vi "BRig_RT_panel_Laser1_DAB_v1,10.vi"(7 "input_setValues":bool, 9 "input_dataExp":u16[](array[numeric]), 11 "input_dataLC":u16[](array[numeric])) -> (1 "output_dataExp":u16[](array[numeric]), 3 "output_dataLC":u16[](array[numeric]))   [LabVIEW 2014]
panel:
  out "LaserPulseTrain":cluster{u16[], u16[]}(graph)
  in  "LED_baseline":bool
  in  "Laser_power_step":dbl
  in  "Laser_power_max":dbl
  in  "Laser_power_min":dbl
  in  "Laser_Tshutter":u16=2
  in  "Laser_Freq":u16=10
  in  "Laser_Tpeak":u16=2
  in  "Laser_T":u16
  in  "LC_Sel_First_Count":u16
  in  "LC_Sel_First_Probability":u16
  in  "LC_Sel_First_Block":u16(slide) max=2 step=1 scale=0.0..2.0
  in  "LC_Sel_First_OnOff":bool
  in  "LC_Sel_First_Tdelay":u16
  in  "LC_Cue_First_Count":u16
  in  "LC_ENL_First_Count":u16
  in  "LC_Cue_First_delayOpt":bool
  in  "LC_ENL_First_delayOpt":bool
  in  "LC_Reward_Probability":u16
  in  "LC_Reward_Block":u16(slide) max=2 step=1 scale=0.0..2.0
  in  "LC_Reward_OnOff":bool
  in  "LC_Cue_First_Probability":u16
  in  "LC_Cue_First_Block":u16(slide) max=2 step=1 scale=0.0..2.0
  in  "LC_Cue_First_OnOff":bool
  in  "LC_ENL_First_Probability":u16 max=100 step=1
  in  "LC_ENL_First_Block":u16(slide) max=2 step=1 scale=0.0..2.0
  in  "LC_Reward_Tdelay":u16
  in  "LC_Cue_First_Tdelay":u16
  in  "LC_ENL_First_Tdelay":u16
  in  "LC_ENL_First_OnOff":bool
  # "Laser1 Control\n                               On/Off      Block        Probability [%]   Delay [ms]                              Count"
  # "Enforced\nNonLick"
  # "from end"
  # "from start"
  # "Cue"
  # "from end"
  # "from start"
  # "Selection"
  # "from start"
  # "Laser1 Parameters"
  # "Laser1 Response\n           On/Off      Response                 Probability %  Delay [ms]"
  # "Frequency\n[Hz]"
  # "Selection\nReward"
  # "Timing [ms]\n Duration     Peak Width   Shutter"
  # "If flip event (reward amount and probability get flipped)\nthen adjust the response setting as well (e.g. Left->Right)"
  # "Laser Power [V]\nMin          Max              Step"
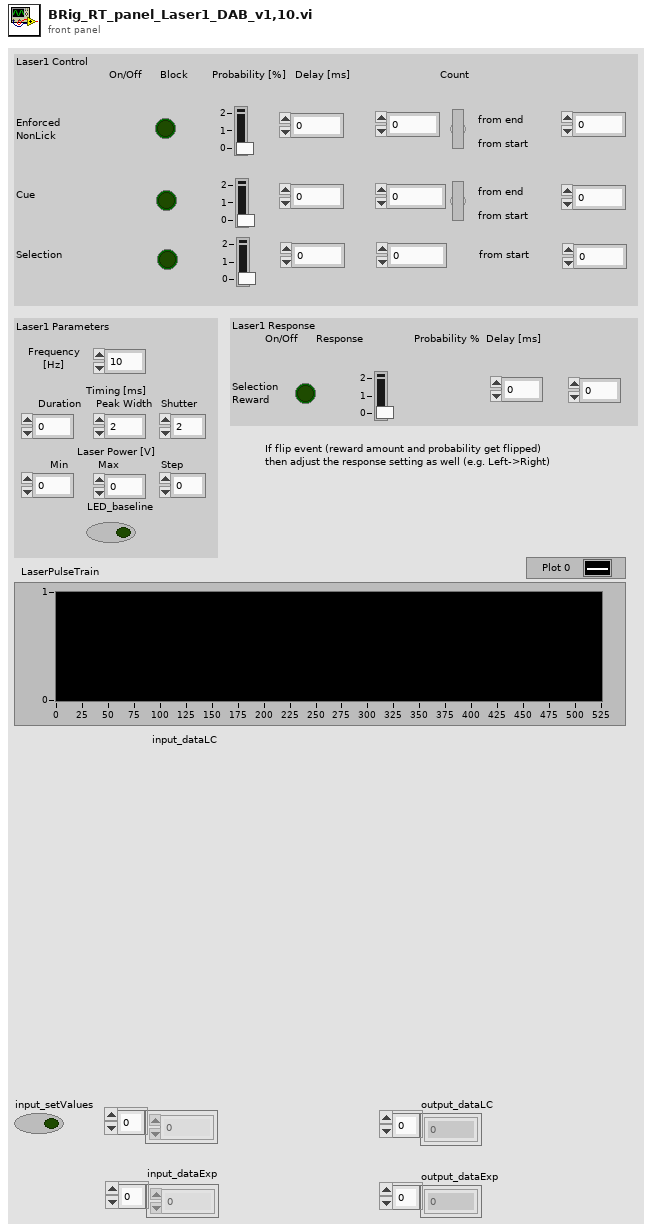
[diagram p1: front panel]
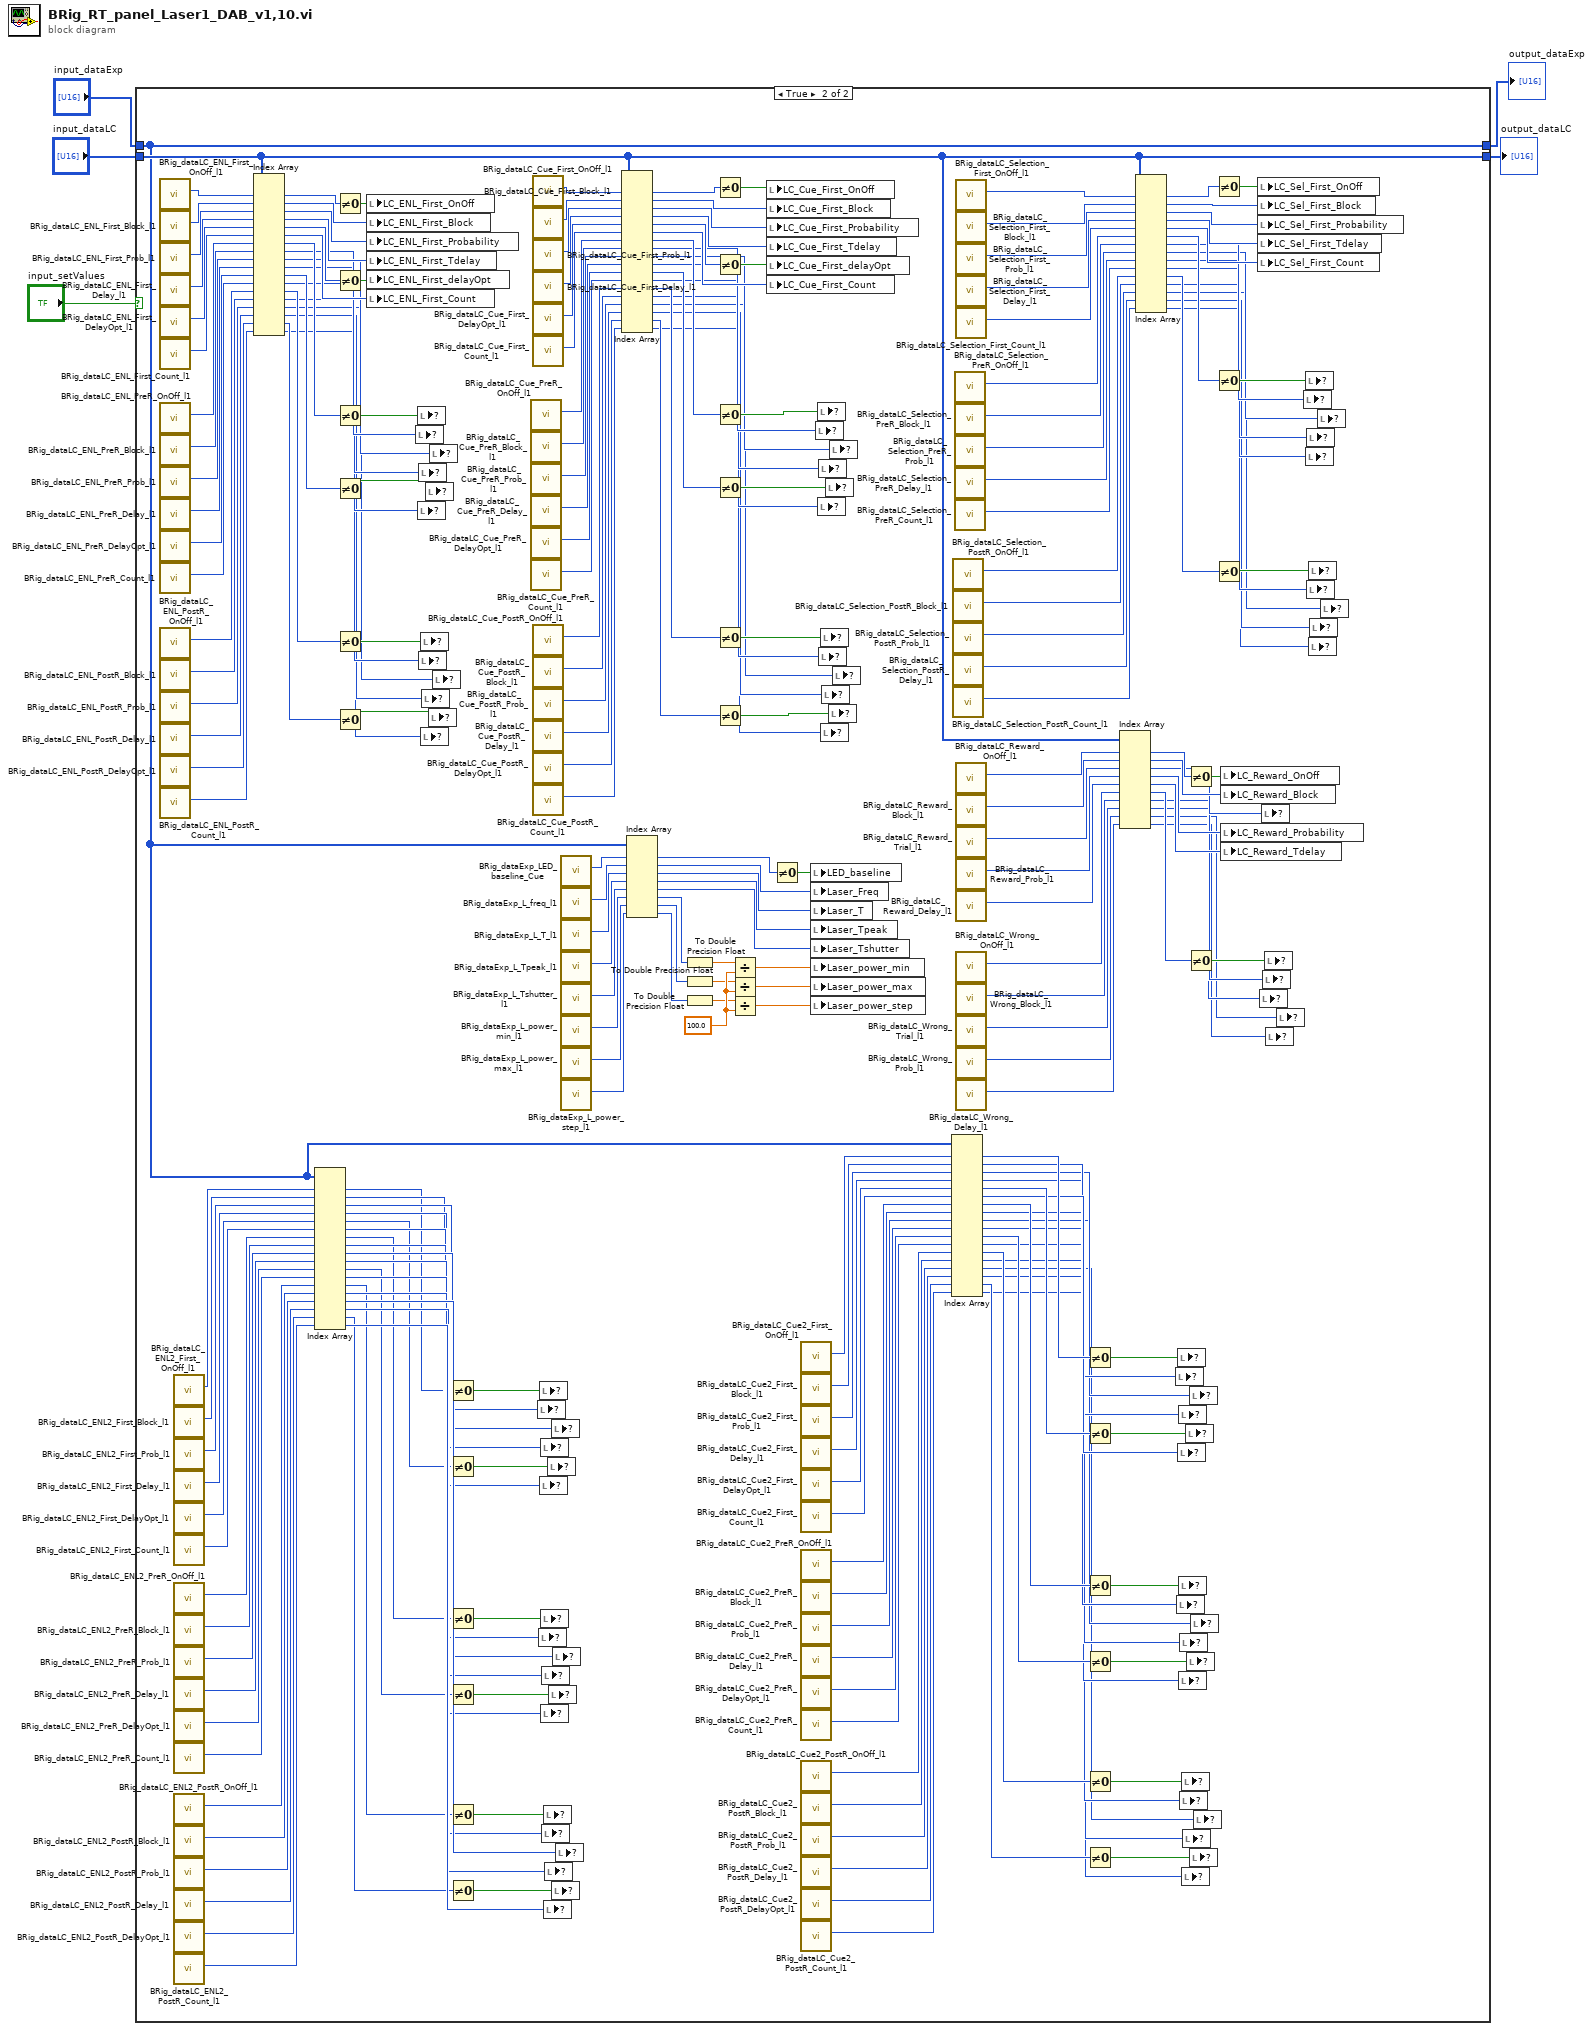
[diagram p0: block diagram]
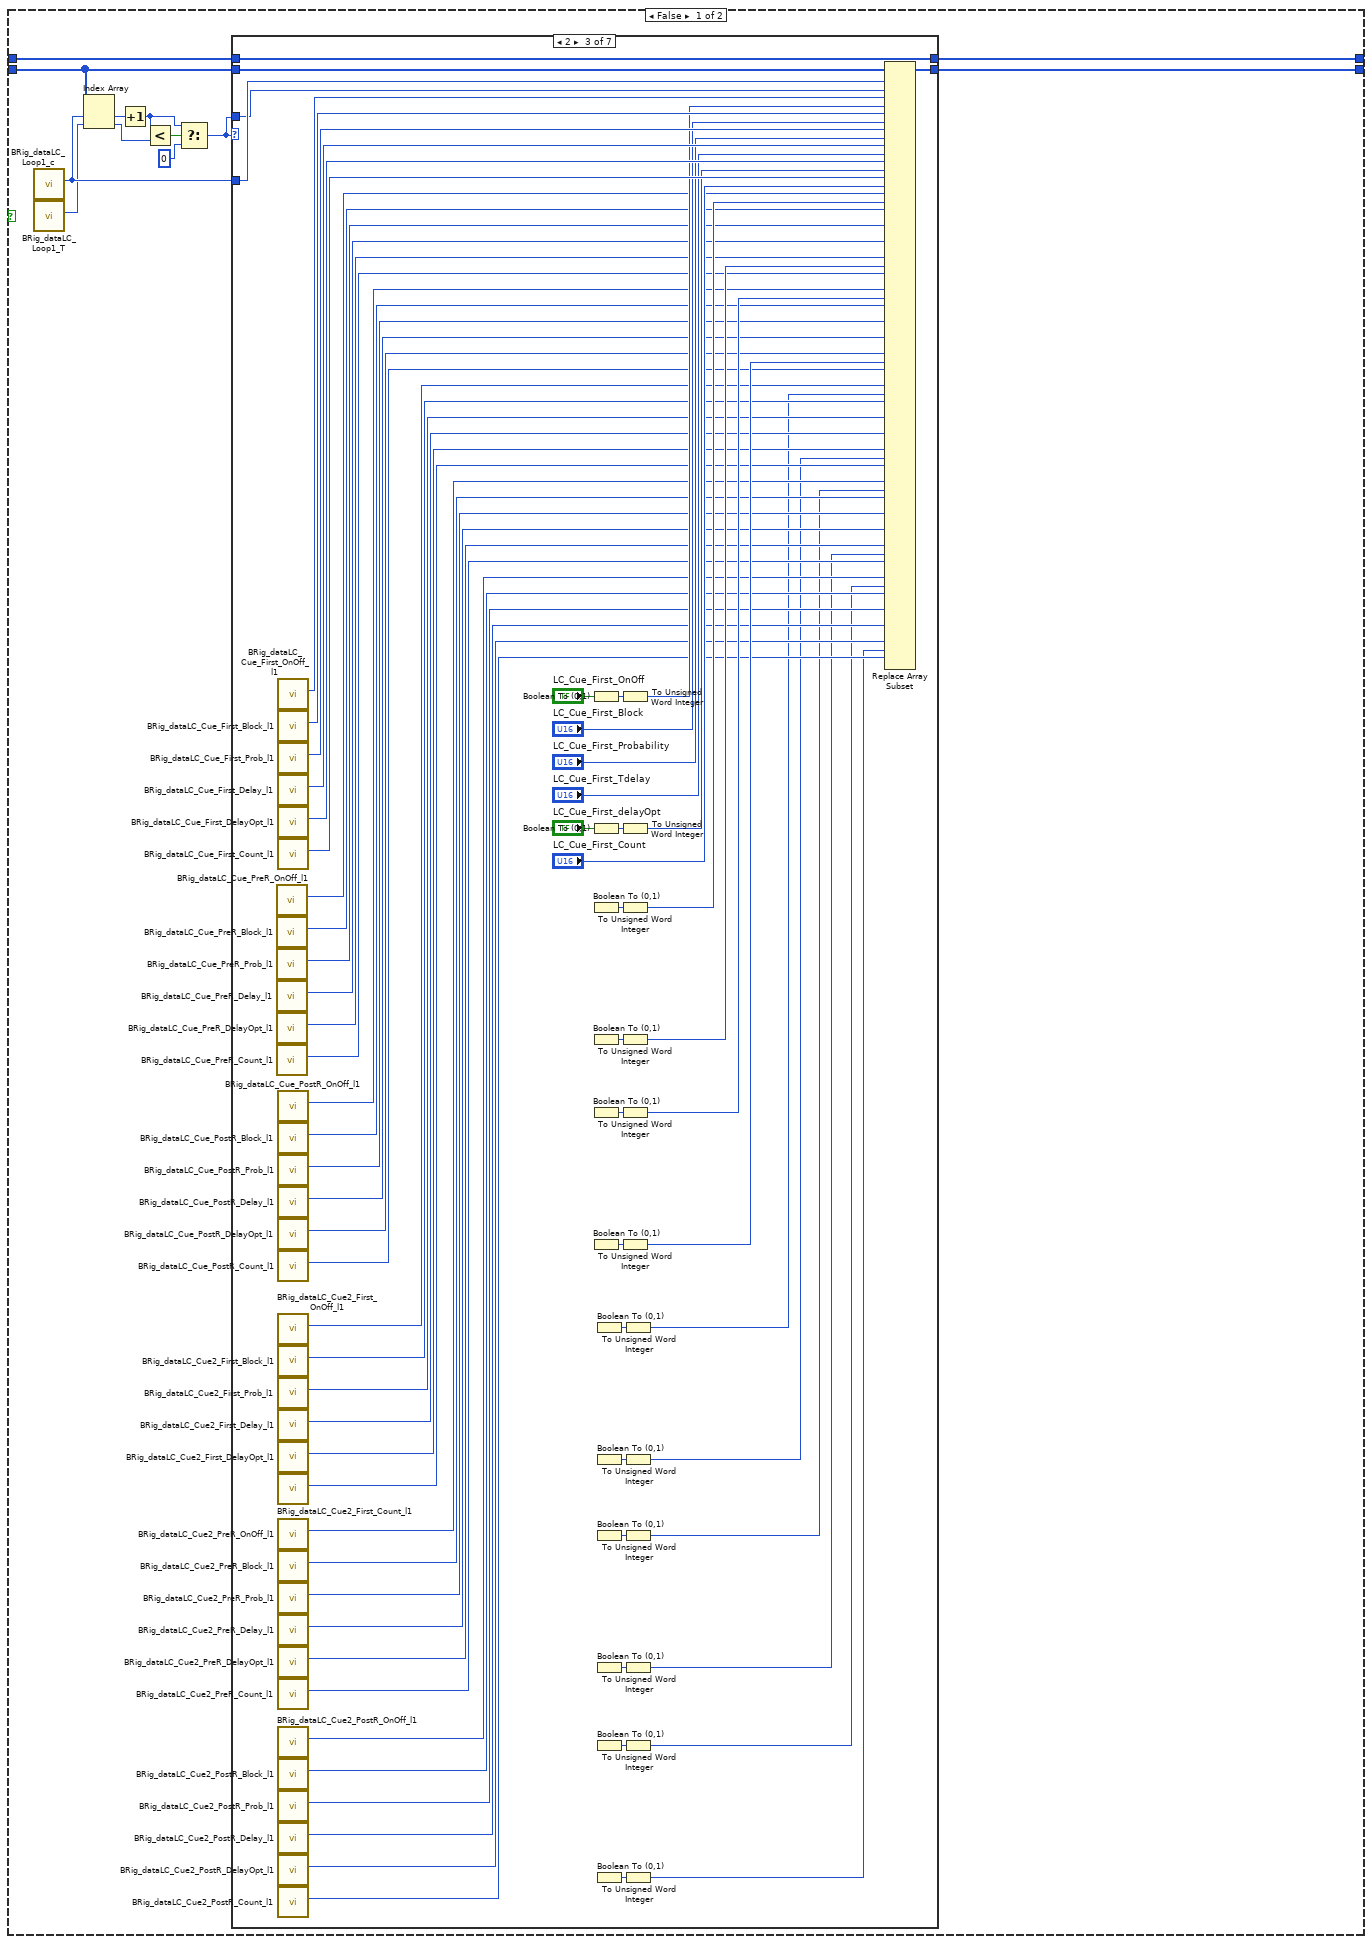
[diagram p2: hidden frame]
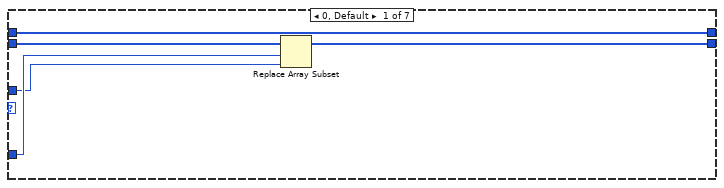
[diagram p3: hidden frame]
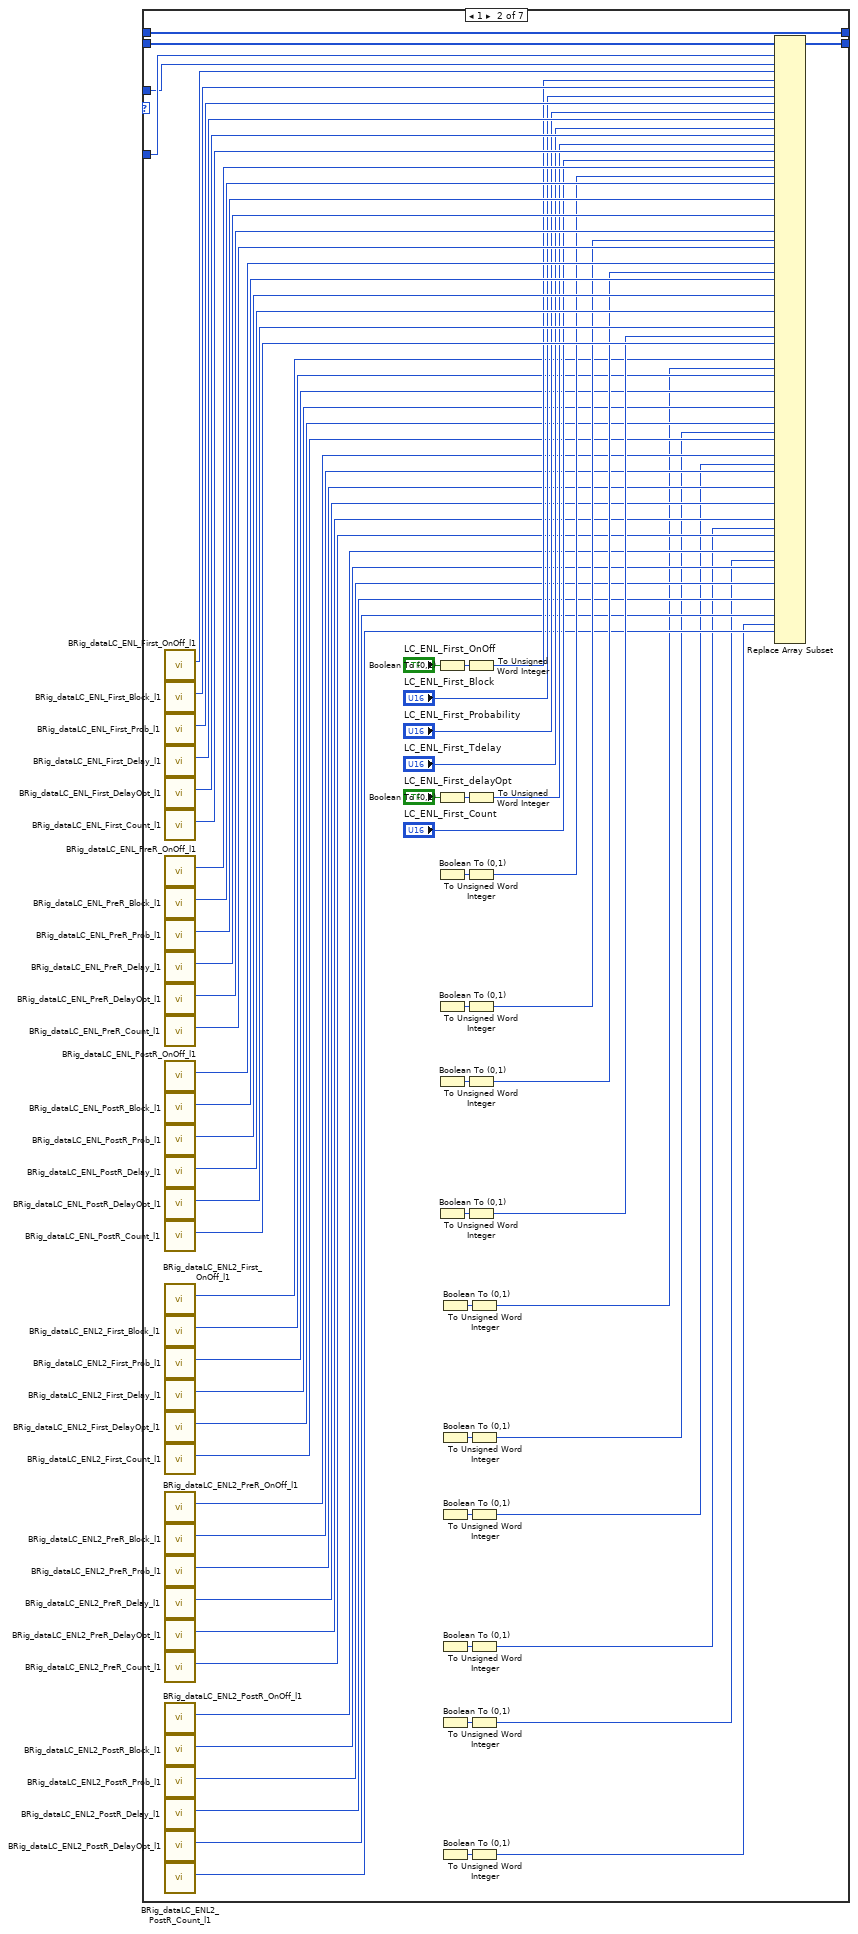
[diagram p4: hidden frame]
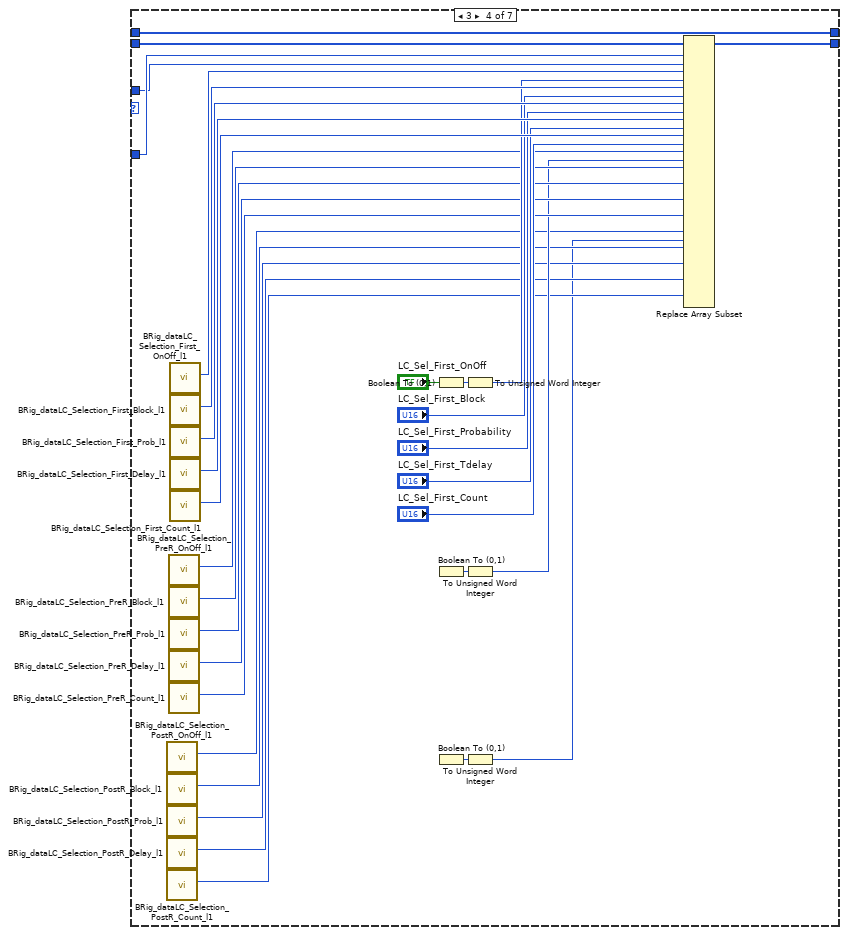
[diagram p5: hidden frame]
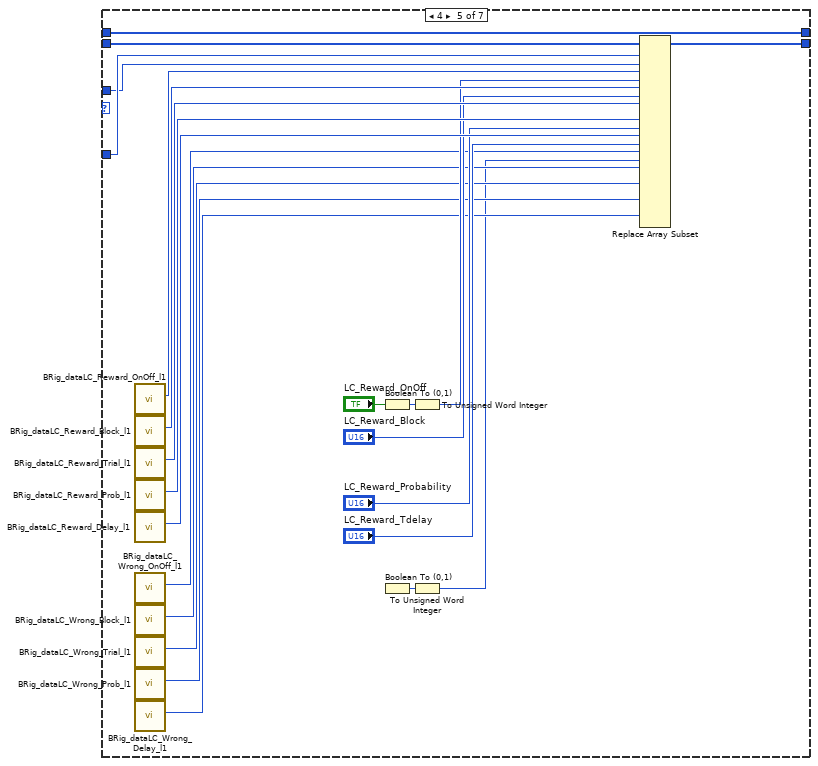
[diagram p6: hidden frame]
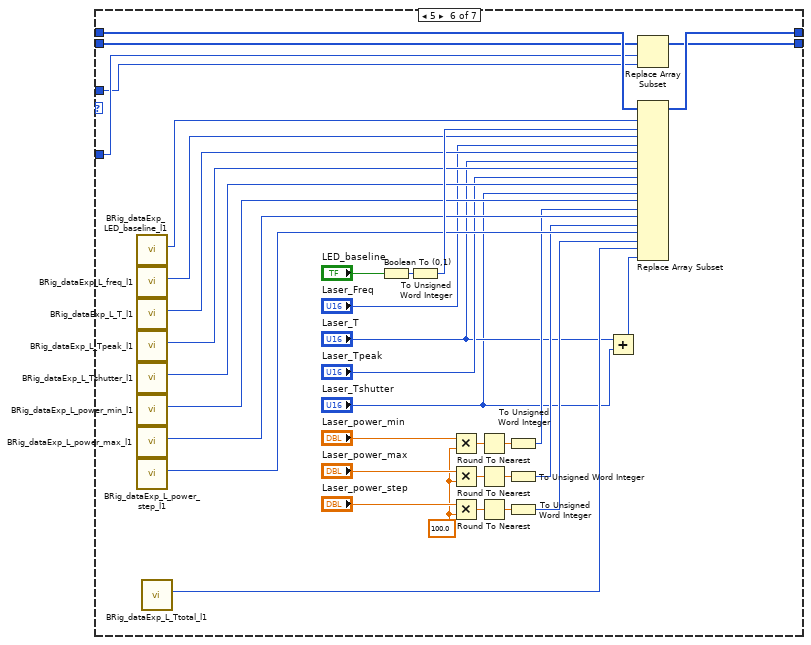
[diagram p7: hidden frame]
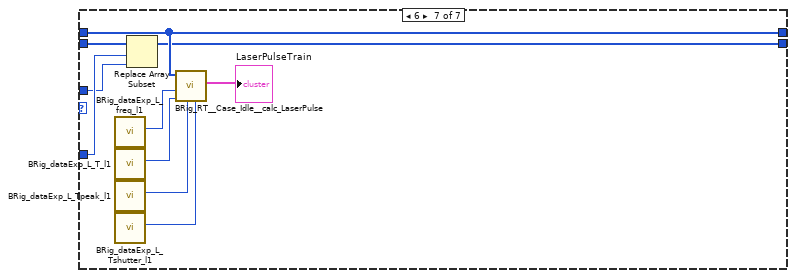
[diagram p8: hidden frame]
diagram:
  n1 = case shown="True" "input_setValues" {
    tunnel: "input_dataLC" -> [w17 w445]
    tunnel: [w11 w445] -> w4
    tunnel: "input_dataExp" -> [w7 w360]
    tunnel: [w6 w360] -> w1
    frame False {
      n2 = call "BRig_dataLC_Loop1_c.vi"() -> ("output_Loop1_c"=w10:i32)  [unwired: 11 in]
      n3 = call "BRig_dataLC_Loop1_T.vi"() -> ("output_Loop1_T"=w9:i32)  [unwired: 11 in]
      n4 = Index Array(array=w17, index #1=w10, index #2=w9) -> (element #1=w16:u16, element #2=w15:u16)
      n5 = Increment(x=w16) -> (x+1=w12:u16)
      n6 = Less?(x=w12, y=w15) -> (x < y?=w14:bool)
      n7 = Select(t=w12, s=w14, f=u16 0) -> (s? t:f=w8:u16)
      n8 = case shown="2" w8 {
        tunnel: w17 -> [w22 w113 w210 w249 w277 w282 w321]
        tunnel: w10 -> [w20 w67 w176 w213 w252 w280 w319]
        tunnel: w8 -> [w19 w66 w175 w212 w251 w279 w318]
        tunnel: [w21 w106 w209 w248 w276 w281 w320] -> w11
        tunnel: w7 -> [w18 w65 w162 w211 w250 w284 w323]
        tunnel: [w18 w65 w162 w211 w250 w283 w323] -> w6
        frame 0, Default {
          n9 = Replace Array Subset(array=w22, new element=w19, index=w20) -> (w21:u16[])
        }
        frame 1 {
          n10 = call "BRig_dataLC_ENL_First_OnOff_l1.vi"() -> ("output_ENL_First_OnOff"=w112:i32)  [unwired: 11 in]
          n11 = call "BRig_dataLC_ENL_First_Block_l1.vi"() -> ("output_ENL_First_Block"=w111:i32)  [unwired: 11 in]
          n12 = call "BRig_dataLC_ENL_First_Prob_l1.vi"() -> ("output_ENL_First_Prob"=w110:i32)  [unwired: 11 in]
          n13 = call "BRig_dataLC_ENL_First_Delay_l1.vi"() -> ("output_ENL_First_Delay"=w109:i32)  [unwired: 11 in]
          n14 = call "BRig_dataLC_ENL_First_DelayOpt_l1.vi"() -> ("output_ENL_First_DelayOpt"=w108:i32)  [unwired: 11 in]
          n15 = call "BRig_dataLC_ENL_First_Count_l1.vi"() -> ("output_ENL_First_Count"=w107:i32)  [unwired: 11 in]
          n16 = call "BRig_dataLC_ENL_PreR_OnOff_l1.vi"() -> ("output_ENL_PreR_OnOff"=w105:i32)  [unwired: 11 in]
          n17 = call "BRig_dataLC_ENL_PreR_Block_l1.vi"() -> ("output_ENL_PreR_Block"=w104:i32)  [unwired: 11 in]
          n18 = call "BRig_dataLC_ENL_PreR_Prob_l1.vi"() -> ("output_ENL_PreR_Prob"=w103:i32)  [unwired: 11 in]
          n19 = call "BRig_dataLC_ENL_PreR_Delay_l1.vi"() -> ("output_ENL_PreR_Delay"=w102:i32)  [unwired: 11 in]
          n20 = call "BRig_dataLC_ENL_PreR_DelayOpt_l1.vi"() -> ("output_ENL_PreR_DelayOpt"=w101:i32)  [unwired: 11 in]
          n21 = call "BRig_dataLC_ENL_PreR_Count_l1.vi"() -> ("output_ENL_PreR_Count"=w100:i32)  [unwired: 11 in]
          n22 = call "BRig_dataLC_ENL_PostR_OnOff_l1.vi"() -> ("output_ENL_PostR_OnOff"=w99:i32)  [unwired: 11 in]
          n23 = call "BRig_dataLC_ENL_PostR_Block_l1.vi"() -> ("output_ENL_PostR_Block"=w98:i32)  [unwired: 11 in]
          n24 = call "BRig_dataLC_ENL_PostR_Prob_l1.vi"() -> ("output_ENL_PostR_Prob"=w97:i32)  [unwired: 11 in]
          n25 = call "BRig_dataLC_ENL_PostR_Delay_l1.vi"() -> ("output_ENL_PostR_Delay"=w96:i32)  [unwired: 11 in]
          n26 = call "BRig_dataLC_ENL_PostR_DelayOpt_l1.vi"() -> ("output_ENL_PostR_DelayOpt"=w95:i32)  [unwired: 11 in]
          n27 = call "BRig_dataLC_ENL_PostR_Count_l1.vi"() -> ("output_ENL_PostR_Count"=w94:i32)  [unwired: 11 in]
          n28 = call "BRig_dataLC_ENL2_First_OnOff_l1.vi"() -> ("output_ENL2_First_OnOff"=w64:i32)  [unwired: 11 in]
          n29 = call "BRig_dataLC_ENL2_First_Block_l1.vi"() -> ("output_ENL2_First_Block"=w63:i32)  [unwired: 11 in]
          n30 = call "BRig_dataLC_ENL2_First_Prob_l1.vi"() -> ("output_ENL2_First_Prob"=w62:i32)  [unwired: 11 in]
          n31 = call "BRig_dataLC_ENL2_First_Delay_l1.vi"() -> ("output_ENL2_First_Delay"=w61:i32)  [unwired: 11 in]
          n32 = call "BRig_dataLC_ENL2_First_DelayOpt_l1.vi"() -> ("output_ENL2_First_DelayOpt"=w60:i32)  [unwired: 11 in]
          n33 = call "BRig_dataLC_ENL2_First_Count_l1.vi"() -> ("output_ENL2_First_Count"=w59:i32)  [unwired: 11 in]
          n34 = call "BRig_dataLC_ENL2_PreR_OnOff_l1.vi"() -> ("output_ENL2_PreR_OnOff"=w58:i32)  [unwired: 11 in]
          n35 = call "BRig_dataLC_ENL2_PreR_Block_l1.vi"() -> ("output_ENL2_PreR_Block"=w57:i32)  [unwired: 11 in]
          n36 = call "BRig_dataLC_ENL2_PreR_Prob_l1.vi"() -> ("output_ENL2_PreR_Prob"=w56:i32)  [unwired: 11 in]
          n37 = call "BRig_dataLC_ENL2_PreR_Delay_l1.vi"() -> ("output_ENL2_PreR_Delay"=w55:i32)  [unwired: 11 in]
          n38 = call "BRig_dataLC_ENL2_PreR_DelayOpt_l1.vi"() -> ("output_ENL2_PreR_DelayOpt"=w54:i32)  [unwired: 11 in]
          n39 = call "BRig_dataLC_ENL2_PreR_Count_l1.vi"() -> ("output_ENL2_PreR_Count"=w53:i32)  [unwired: 11 in]
          n40 = call "BRig_dataLC_ENL2_PostR_OnOff_l1.vi"() -> ("output_ENL2_PostR_OnOff"=w52:i32)  [unwired: 11 in]
          n41 = call "BRig_dataLC_ENL2_PostR_Block_l1.vi"() -> ("output_ENL2_PostR_Block"=w51:i32)  [unwired: 11 in]
          n42 = call "BRig_dataLC_ENL2_PostR_Prob_l1.vi"() -> ("output_ENL2_PostR_Prob"=w50:i32)  [unwired: 11 in]
          n43 = call "BRig_dataLC_ENL2_PostR_Delay_l1.vi"() -> ("output_ENL2_PostR_Delay"=w49:i32)  [unwired: 11 in]
          n44 = call "BRig_dataLC_ENL2_PostR_DelayOpt_l1.vi"() -> ("output_ENL2_PostR_DelayOpt"=w48:i32)  [unwired: 11 in]
          n45 = call "BRig_dataLC_ENL2_PostR_Count_l1.vi"() -> ("output_ENL2_PostR_Count"=w47:i32)  [unwired: 11 in]
          n46 = Boolean To (0,1)(Boolean="LC_ENL_First_OnOff") -> (0, 1=w92:i16)
          n47 = Boolean To (0,1)(Boolean="LC_ENL_First_delayOpt") -> (0, 1=w91:i16)
          n48 = Boolean To (0,1)() -> (0, 1=w89:i16)  [unwired: 1 in]
          n49 = Boolean To (0,1)() -> (0, 1=w88:i16)  [unwired: 1 in]
          n50 = Boolean To (0,1)() -> (0, 1=w87:i16)  [unwired: 1 in]
          n51 = Boolean To (0,1)() -> (0, 1=w86:i16)  [unwired: 1 in]
          n52 = Boolean To (0,1)() -> (0, 1=w39:i16)  [unwired: 1 in]
          n53 = Boolean To (0,1)() -> (0, 1=w38:i16)  [unwired: 1 in]
          n54 = Boolean To (0,1)() -> (0, 1=w37:i16)  [unwired: 1 in]
          n55 = Boolean To (0,1)() -> (0, 1=w36:i16)  [unwired: 1 in]
          n56 = Boolean To (0,1)() -> (0, 1=w29:i16)  [unwired: 1 in]
          n57 = Boolean To (0,1)() -> (0, 1=w28:i16)  [unwired: 1 in]
          n58 = To Unsigned Word Integer(number=w92) -> (unsigned 16bit integer=w85:u16)
          n59 = To Unsigned Word Integer(number=w91) -> (unsigned 16bit integer=w81:u16)
          n60 = To Unsigned Word Integer(number=w89) -> (unsigned 16bit integer=w79:u16)
          n61 = To Unsigned Word Integer(number=w88) -> (unsigned 16bit integer=w75:u16)
          n62 = To Unsigned Word Integer(number=w87) -> (unsigned 16bit integer=w73:u16)
          n63 = To Unsigned Word Integer(number=w86) -> (unsigned 16bit integer=w69:u16)
          n64 = To Unsigned Word Integer(number=w39) -> (unsigned 16bit integer=w46:u16)
          n65 = To Unsigned Word Integer(number=w38) -> (unsigned 16bit integer=w42:u16)
          n66 = To Unsigned Word Integer(number=w37) -> (unsigned 16bit integer=w40:u16)
          n67 = To Unsigned Word Integer(number=w36) -> (unsigned 16bit integer=w32:u16)
          n68 = To Unsigned Word Integer(number=w29) -> (unsigned 16bit integer=w30:u16)
          n69 = To Unsigned Word Integer(number=w28) -> (unsigned 16bit integer=w24:u16)
          n70 = Replace Array Subset(array=w113, new element #1=w66, index #1=w67, new element #2=w85, index #2=w112, new element #3="LC_ENL_First_Block", index #3=w111, new element #4="LC_ENL_First_Probability", index #4=w110, new element #5="LC_ENL_First_Tdelay", index #5=w109, new element #6=w81, index #6=w108, new element #7="LC_ENL_First_Count", index #7=w107, new element #8=w79, index #8=w105, index #9=w104, index #10=w103, index #11=w102, new element #12=w75, index #12=w101, index #13=w100, new element #14=w73, index #14=w99, index #15=w98, index #16=w97, index #17=w96, new element #18=w69, index #18=w95, index #19=w94, new element #20=w46, index #20=w64, index #21=w63, index #22=w62, index #23=w61, new element #24=w42, index #24=w60, index #25=w59, new element #26=w40, index #26=w58, index #27=w57, index #28=w56, index #29=w55, new element #30=w32, index #30=w54, index #31=w53, new element #32=w30, index #32=w52, index #33=w51, index #34=w50, index #35=w49, new element #36=w24, index #36=w48, index #37=w47) -> (w106:u16[], new element #9=w78:u16, new element #10=w77:u16, new element #11=w76:u16, new element #13=w74:u16, new element #15=w72:u16, new element #16=w71:u16, new element #17=w70:u16, new element #19=w68:u16, new element #21=w45:u16, new element #22=w44:u16, new element #23=w43:u16, new element #25=w41:u16, new element #27=w35:u16, new element #28=w34:u16, new element #29=w33:u16, new element #31=w31:u16, new element #33=w27:u16, new element #34=w26:u16, new element #35=w25:u16, new element #37=w23:u16)
        }
        frame 2 {
          n71 = call "BRig_dataLC_Cue_PreR_OnOff_l1.vi"() -> ("output_Cue_PreR_OnOff"=w172:i32)  [unwired: 11 in]
          n72 = call "BRig_dataLC_Cue_PreR_Block_l1.vi"() -> ("output_Cue_PreR_Block"=w171:i32)  [unwired: 11 in]
          n73 = call "BRig_dataLC_Cue_PreR_Prob_l1.vi"() -> ("output_Cue_PreR_Prob"=w170:i32)  [unwired: 11 in]
          n74 = call "BRig_dataLC_Cue_PreR_Delay_l1.vi"() -> ("output_Cue_PreR_Delay"=w169:i32)  [unwired: 11 in]
          n75 = call "BRig_dataLC_Cue_PreR_DelayOpt_l1.vi"() -> ("output_Cue_PreR_DelayOpt"=w168:i32)  [unwired: 11 in]
          n76 = call "BRig_dataLC_Cue_PreR_Count_l1.vi"() -> ("output_Cue_PreR_Count"=w173:i32)  [unwired: 11 in]
          n77 = call "BRig_dataLC_Cue_First_OnOff_l1.vi"() -> ("output_Cue_First_OnOff"=w208:i32)  [unwired: 11 in]
          n78 = call "BRig_dataLC_Cue_First_Block_l1.vi"() -> ("output_Cue_First_Block"=w207:i32)  [unwired: 11 in]
          n79 = call "BRig_dataLC_Cue_First_Prob_l1.vi"() -> ("output_Cue_First_Prob"=w206:i32)  [unwired: 11 in]
          n80 = call "BRig_dataLC_Cue_First_Delay_l1.vi"() -> ("output_Cue_First_Delay"=w205:i32)  [unwired: 11 in]
          n81 = call "BRig_dataLC_Cue_First_DelayOpt_l1.vi"() -> ("output_Cue_First_DelayOpt"=w204:i32)  [unwired: 11 in]
          n82 = call "BRig_dataLC_Cue_First_Count_l1.vi"() -> ("output_Cue_First_Count"=w203:i32)  [unwired: 11 in]
          n83 = call "BRig_dataLC_Cue_PostR_OnOff_l1.vi"() -> ("output_Cue_PostR_OnOff"=w174:i32)  [unwired: 11 in]
          n84 = call "BRig_dataLC_Cue_PostR_Block_l1.vi"() -> ("output_Cue_PostR_Block"=w167:i32)  [unwired: 11 in]
          n85 = call "BRig_dataLC_Cue_PostR_Prob_l1.vi"() -> ("output_Cue_PostR_Prob"=w166:i32)  [unwired: 11 in]
          n86 = call "BRig_dataLC_Cue_PostR_Delay_l1.vi"() -> ("output_Cue_PostR_Delay"=w165:i32)  [unwired: 11 in]
          n87 = call "BRig_dataLC_Cue_PostR_DelayOpt_l1.vi"() -> ("output_Cue_PostR_DelayOpt"=w164:i32)  [unwired: 11 in]
          n88 = call "BRig_dataLC_Cue_PostR_Count_l1.vi"() -> ("output_Cue_PostR_Count"=w163:i32)  [unwired: 11 in]
          n89 = call "BRig_dataLC_Cue2_First_OnOff_l1.vi"() -> ("output_Cue2_First_OnOff"=w161:i32)  [unwired: 11 in]
          n90 = call "BRig_dataLC_Cue2_First_Block_l1.vi"() -> ("output_Cue2_First_Block"=w160:i32)  [unwired: 11 in]
          n91 = call "BRig_dataLC_Cue2_First_Prob_l1.vi"() -> ("output_Cue2_First_Prob"=w159:i32)  [unwired: 11 in]
          n92 = call "BRig_dataLC_Cue2_First_Delay_l1.vi"() -> ("output_Cue2_First_Delay"=w158:i32)  [unwired: 11 in]
          n93 = call "BRig_dataLC_Cue2_First_DelayOpt_l1.vi"() -> ("output_Cue2_First_DelayOpt"=w157:i32)  [unwired: 11 in]
          n94 = call "BRig_dataLC_Cue2_First_Count_l1.vi"() -> ("output_Cue2_First_Count"=w156:i32)  [unwired: 11 in]
          n95 = call "BRig_dataLC_Cue2_PreR_OnOff_l1.vi"() -> ("output_Cue2_PreR_OnOff"=w155:i32)  [unwired: 11 in]
          n96 = call "BRig_dataLC_Cue2_PreR_Block_l1.vi"() -> ("output_Cue2_PreR_Block"=w154:i32)  [unwired: 11 in]
          n97 = call "BRig_dataLC_Cue2_PreR_Prob_l1.vi"() -> ("output_Cue2_PreR_Prob"=w153:i32)  [unwired: 11 in]
          n98 = call "BRig_dataLC_Cue2_PreR_Delay_l1.vi"() -> ("output_Cue2_PreR_Delay"=w152:i32)  [unwired: 11 in]
          n99 = call "BRig_dataLC_Cue2_PreR_DelayOpt_l1.vi"() -> ("output_Cue2_PreR_DelayOpt"=w151:i32)  [unwired: 11 in]
          n100 = call "BRig_dataLC_Cue2_PreR_Count_l1.vi"() -> ("output_Cue2_PreR_Count"=w150:i32)  [unwired: 11 in]
          n101 = call "BRig_dataLC_Cue2_PostR_OnOff_l1.vi"() -> ("output_Cue2_PostR_OnOff"=w149:i32)  [unwired: 11 in]
          n102 = call "BRig_dataLC_Cue2_PostR_Block_l1.vi"() -> ("output_Cue2_PostR_Block"=w148:i32)  [unwired: 11 in]
          n103 = call "BRig_dataLC_Cue2_PostR_Prob_l1.vi"() -> ("output_Cue2_PostR_Prob"=w147:i32)  [unwired: 11 in]
          n104 = call "BRig_dataLC_Cue2_PostR_Delay_l1.vi"() -> ("output_Cue2_PostR_Delay"=w146:i32)  [unwired: 11 in]
          n105 = call "BRig_dataLC_Cue2_PostR_DelayOpt_l1.vi"() -> ("output_Cue2_PostR_DelayOpt"=w145:i32)  [unwired: 11 in]
          n106 = call "BRig_dataLC_Cue2_PostR_Count_l1.vi"() -> ("output_Cue2_PostR_Count"=w144:i32)  [unwired: 11 in]
          n107 = Boolean To (0,1)(Boolean="LC_Cue_First_OnOff") -> (0, 1=w200:i16)
          n108 = Boolean To (0,1)(Boolean="LC_Cue_First_delayOpt") -> (0, 1=w199:i16)
          n109 = Boolean To (0,1)() -> (0, 1=w198:i16)  [unwired: 1 in]
          n110 = Boolean To (0,1)() -> (0, 1=w197:i16)  [unwired: 1 in]
          n111 = Boolean To (0,1)() -> (0, 1=w196:i16)  [unwired: 1 in]
          n112 = Boolean To (0,1)() -> (0, 1=w195:i16)  [unwired: 1 in]
          n113 = Boolean To (0,1)() -> (Boolean=w137:bool, 0, 1=w143:i16)
          n114 = Boolean To (0,1)() -> (Boolean=w136:bool, 0, 1=w142:i16)
          n115 = Boolean To (0,1)() -> (Boolean=w135:bool, 0, 1=w141:i16)
          n116 = Boolean To (0,1)() -> (Boolean=w134:bool, 0, 1=w140:i16)
          n117 = Boolean To (0,1)() -> (Boolean=w133:bool, 0, 1=w139:i16)
          n118 = Boolean To (0,1)() -> (Boolean=w132:bool, 0, 1=w138:i16)
          n119 = To Unsigned Word Integer(number=w200) -> (unsigned 16bit integer=w194:u16)
          n120 = To Unsigned Word Integer(number=w199) -> (unsigned 16bit integer=w190:u16)
          n121 = To Unsigned Word Integer(number=w198) -> (unsigned 16bit integer=w188:u16)
          n122 = To Unsigned Word Integer(number=w197) -> (unsigned 16bit integer=w184:u16)
          n123 = To Unsigned Word Integer(number=w196) -> (unsigned 16bit integer=w182:u16)
          n124 = To Unsigned Word Integer(number=w195) -> (unsigned 16bit integer=w178:u16)
          n125 = To Unsigned Word Integer(number=w143) -> (unsigned 16bit integer=w131:u16)
          n126 = To Unsigned Word Integer(number=w142) -> (unsigned 16bit integer=w127:u16)
          n127 = To Unsigned Word Integer(number=w141) -> (unsigned 16bit integer=w125:u16)
          n128 = To Unsigned Word Integer(number=w140) -> (unsigned 16bit integer=w121:u16)
          n129 = To Unsigned Word Integer(number=w139) -> (unsigned 16bit integer=w119:u16)
          n130 = To Unsigned Word Integer(number=w138) -> (unsigned 16bit integer=w115:u16)
          n131 = Replace Array Subset(array=w210, new element #1=w175, index #1=w176, new element #2=w194, index #2=w208, new element #3="LC_Cue_First_Block", index #3=w207, new element #4="LC_Cue_First_Probability", index #4=w206, new element #5="LC_Cue_First_Tdelay", index #5=w205, new element #6=w190, index #6=w204, new element #7="LC_Cue_First_Count", index #7=w203, new element #8=w188, index #8=w172, index #9=w171, index #10=w170, index #11=w169, new element #12=w184, index #12=w168, index #13=w173, new element #14=w182, index #14=w174, index #15=w167, index #16=w166, index #17=w165, new element #18=w178, index #18=w164, index #19=w163, new element #20=w131, index #20=w161, index #21=w160, index #22=w159, index #23=w158, new element #24=w127, index #24=w157, index #25=w156, new element #26=w125, index #26=w155, index #27=w154, index #28=w153, index #29=w152, new element #30=w121, index #30=w151, index #31=w150, new element #32=w119, index #32=w149, index #33=w148, index #34=w147, index #35=w146, new element #36=w115, index #36=w145, index #37=w144) -> (w209:u16[], new element #9=w187:u16, new element #10=w186:u16, new element #11=w185:u16, new element #13=w183:u16, new element #15=w181:u16, new element #16=w180:u16, new element #17=w179:u16, new element #19=w177:u16, new element #21=w130:u16, new element #22=w129:u16, new element #23=w128:u16, new element #25=w126:u16, new element #27=w124:u16, new element #28=w123:u16, new element #29=w122:u16, new element #31=w120:u16, new element #33=w118:u16, new element #34=w117:u16, new element #35=w116:u16, new element #37=w114:u16)
        }
        frame 3 {
          n132 = call "BRig_dataLC_Selection_PostR_OnOff_l1.vi"() -> ("output_Selection_PostR_OnOff"=w223:i32)  [unwired: 11 in]
          n133 = call "BRig_dataLC_Selection_PostR_Block_l1.vi"() -> ("output_Selection_PostR_Block"=w222:i32)  [unwired: 11 in]
          n134 = call "BRig_dataLC_Selection_PostR_Prob_l1.vi"() -> ("output_Selection_PostR_Prob"=w221:i32)  [unwired: 11 in]
          n135 = call "BRig_dataLC_Selection_PostR_Delay_l1.vi"() -> ("output_Selection_PostR_Delay"=w220:i32)  [unwired: 11 in]
          n136 = call "BRig_dataLC_Selection_PostR_Count_l1.vi"() -> ("output_Selection_PostR_Count"=w219:i32)  [unwired: 11 in]
          n137 = call "BRig_dataLC_Selection_PreR_OnOff_l1.vi"() -> ("output_Selection_PreR_OnOff"=w233:i32)  [unwired: 11 in]
          n138 = call "BRig_dataLC_Selection_PreR_Block_l1.vi"() -> ("output_Selection_PreR_Block"=w232:i32)  [unwired: 11 in]
          n139 = call "BRig_dataLC_Selection_PreR_Prob_l1.vi"() -> ("output_Selection_PreR_Prob"=w231:i32)  [unwired: 11 in]
          n140 = call "BRig_dataLC_Selection_PreR_Delay_l1.vi"() -> ("output_Selection_PreR_Delay"=w230:i32)  [unwired: 11 in]
          n141 = call "BRig_dataLC_Selection_PreR_Count_l1.vi"() -> ("output_Selection_PreR_Count"=w229:i32)  [unwired: 11 in]
          n142 = call "BRig_dataLC_Selection_First_OnOff_l1.vi"() -> ("output_Selection_First_OnOff"=w243:i32)  [unwired: 11 in]
          n143 = call "BRig_dataLC_Selection_First_Block_l1.vi"() -> ("output_Selection_First_Block"=w242:i32)  [unwired: 11 in]
          n144 = call "BRig_dataLC_Selection_First_Prob_l1.vi"() -> ("output_Selection_First_Prob"=w241:i32)  [unwired: 11 in]
          n145 = call "BRig_dataLC_Selection_First_Delay_l1.vi"() -> ("output_Selection_First_Delay"=w240:i32)  [unwired: 11 in]
          n146 = call "BRig_dataLC_Selection_First_Count_l1.vi"() -> ("output_Selection_First_Count"=w239:i32)  [unwired: 11 in]
          n147 = Boolean To (0,1)(Boolean="LC_Sel_First_OnOff") -> (0, 1=w246:i16)
          n148 = Boolean To (0,1)() -> (0, 1=w245:i16)  [unwired: 1 in]
          n149 = Boolean To (0,1)() -> (0, 1=w244:i16)  [unwired: 1 in]
          n150 = To Unsigned Word Integer(number=w246) -> (unsigned 16bit integer=w238:u16)
          n151 = To Unsigned Word Integer(number=w245) -> (unsigned 16bit integer=w228:u16)
          n152 = To Unsigned Word Integer(number=w244) -> (unsigned 16bit integer=w218:u16)
          n153 = Replace Array Subset(array=w249, new element #1=w212, index #1=w213, new element #2=w238, index #2=w243, new element #3="LC_Sel_First_Block", index #3=w242, new element #4="LC_Sel_First_Probability", index #4=w241, new element #5="LC_Sel_First_Tdelay", index #5=w240, new element #6="LC_Sel_First_Count", index #6=w239, new element #7=w228, index #7=w233, index #8=w232, index #9=w231, index #10=w230, index #11=w229, new element #12=w218, index #12=w223, index #13=w222, index #14=w221, index #15=w220, index #16=w219) -> (w248:u16[], new element #8=w227:u16, new element #9=w226:u16, new element #10=w225:u16, new element #11=w224:u16, new element #13=w217:u16, new element #14=w216:u16, new element #15=w215:u16, new element #16=w214:u16)
        }
        frame 4 {
          n154 = call "BRig_dataLC_Reward_OnOff_l1.vi"() -> ("output_Reward_OnOff"=w275:i32)  [unwired: 11 in]
          n155 = call "BRig_dataLC_Reward_Block_l1.vi"() -> ("output_Reward_Block"=w274:i32)  [unwired: 11 in]
          n156 = call "BRig_dataLC_Reward_Trial_l1.vi"() -> ("output_Reward_Trial"=w273:i32)  [unwired: 11 in]
          n157 = call "BRig_dataLC_Reward_Prob_l1.vi"() -> ("output_Reward_Prob"=w272:i32)  [unwired: 11 in]
          n158 = call "BRig_dataLC_Reward_Delay_l1.vi"() -> ("output_Reward_Delay"=w271:i32)  [unwired: 11 in]
          n159 = call "BRig_dataLC_Wrong_OnOff_l1.vi"() -> ("output_Wrong_OnOff"=w262:i32)  [unwired: 11 in]
          n160 = call "BRig_dataLC_Wrong_Block_l1.vi"() -> ("output_Wrong_Block"=w261:i32)  [unwired: 11 in]
          n161 = call "BRig_dataLC_Wrong_Trial_l1.vi"() -> ("output_Wrong_Trial"=w260:i32)  [unwired: 11 in]
          n162 = call "BRig_dataLC_Wrong_Prob_l1.vi"() -> ("output_Wrong_Prob"=w259:i32)  [unwired: 11 in]
          n163 = call "BRig_dataLC_Wrong_Delay_l1.vi"() -> ("output_Wrong_Delay"=w258:i32)  [unwired: 11 in]
          n164 = Boolean To (0,1)(Boolean="LC_Reward_OnOff") -> (0, 1=w269:i16)
          n165 = Boolean To (0,1)() -> (0, 1=w268:i16)  [unwired: 1 in]
          n166 = To Unsigned Word Integer(number=w269) -> (unsigned 16bit integer=w267:u16)
          n167 = To Unsigned Word Integer(number=w268) -> (unsigned 16bit integer=w257:u16)
          n168 = Replace Array Subset(array=w277, new element #1=w251, index #1=w252, new element #2=w267, index #2=w275, new element #3="LC_Reward_Block", index #3=w274, index #4=w273, new element #5="LC_Reward_Probability", index #5=w272, new element #6="LC_Reward_Tdelay", index #6=w271, new element #7=w257, index #7=w262, index #8=w261, index #9=w260, index #10=w259, index #11=w258) -> (w276:u16[], new element #4=w265:u16, new element #8=w256:u16, new element #9=w255:u16, new element #10=w254:u16, new element #11=w253:u16)
        }
        frame 5 {
          w301 = 100.0 ("y")
          n169 = call "BRig_dataExp_LED_baseline_l1.vi"() -> ("output_LED_baseline_l1"=w278:i32)  [unwired: 11 in]
          n170 = call "BRig_dataExp_L_freq_l1.vi"() -> ("output_L_freq_l1"=w300:i32)  [unwired: 11 in]
          n171 = call "BRig_dataExp_L_T_l1.vi"() -> ("output_L_T_l1"=w299:i32)  [unwired: 11 in]
          n172 = call "BRig_dataExp_L_Tpeak_l1.vi"() -> ("output_L_Tpeak_l1"=w298:i32)  [unwired: 11 in]
          n173 = call "BRig_dataExp_L_Tshutter_l1.vi"() -> ("output_L_Tshutter_l1"=w297:i32)  [unwired: 11 in]
          n174 = call "BRig_dataExp_L_power_min_l1.vi"() -> ("output_L_power_min_l1"=w296:i32)  [unwired: 11 in]
          n175 = call "BRig_dataExp_L_power_max_l1.vi"() -> ("output_L_power_max_l1"=w295:i32)  [unwired: 11 in]
          n176 = call "BRig_dataExp_L_power_step_l1.vi"() -> ("output_L_power_step_l1"=w294:i32)  [unwired: 11 in]
          n177 = call "BRig_dataExp_L_Ttotal_l1.vi"() -> ("output_L_Ttotal_l1"=w288:i32)  [unwired: 11 in]
          n178 = Boolean To (0,1)(Boolean="LED_baseline") -> (0, 1=w313:i16)
          n179 = To Unsigned Word Integer(number=w313) -> (unsigned 16bit integer=w311:u16)
          n180 = Multiply(x="Laser_power_min", y=w301) -> (x*y=w305:dbl)
          n181 = Multiply(x="Laser_power_max", y=w301) -> (x*y=w307:dbl)
          n182 = Multiply(x="Laser_power_step", y=w301) -> (x*y=w310:dbl)
          n183 = Round To Nearest(number=w305) -> (nearest integer value=w304:dbl)
          n184 = Round To Nearest(number=w307) -> (nearest integer value=w306:dbl)
          n185 = Round To Nearest(number=w310) -> (nearest integer value=w309:dbl)
          n186 = To Unsigned Word Integer(number=w304) -> (unsigned 16bit integer=w291:u16)
          n187 = To Unsigned Word Integer(number=w306) -> (unsigned 16bit integer=w292:u16)
          n188 = To Unsigned Word Integer(number=w309) -> (unsigned 16bit integer=w293:u16)
          n189 = Add(x="Laser_T", y="Laser_Tshutter") -> (x+y=w285:u16)
          n190 = Replace Array Subset(array=w282, new element=w279, index=w280) -> (w281:u16[])
          n191 = Replace Array Subset(array=w284, new element #1=w311, index #1=w278, new element #2="Laser_Freq", index #2=w300, new element #3="Laser_T", index #3=w299, new element #4="Laser_Tpeak", index #4=w298, new element #5="Laser_Tshutter", index #5=w297, new element #6=w291, index #6=w296, new element #7=w292, index #7=w295, new element #8=w293, index #8=w294, new element #9=w285, index #9=w288) -> (w283:u16[])
        }
        frame 6 {
          n192 = call "BRig_dataExp_L_freq_l1.vi"() -> ("output_L_freq_l1"=w316:i32)  [unwired: 11 in]
          n193 = call "BRig_dataExp_L_T_l1.vi"() -> ("output_L_T_l1"=w317:i32)  [unwired: 11 in]
          n194 = call "BRig_dataExp_L_Tpeak_l1.vi"() -> ("output_L_Tpeak_l1"=w315:i32)  [unwired: 11 in]
          n195 = call "BRig_dataExp_L_Tshutter_l1.vi"() -> ("output_L_Tshutter_l1"=w314:i32)  [unwired: 11 in]
          n196 = Replace Array Subset(array=w321, new element=w318, index=w319) -> (w320:u16[])
          n197 = call "BRig_RT__Case_Idle__calc_LaserPulse.vi"("input_dataExp_L_Tshutter"=w314, "input_dataExp_L_Tpeak"=w315, "input_dataExp_L_T"=w317, "input_dataExp_L_freq"=w316, "input_dataExp"=w323) -> ("output_cluster"=→"LaserPulseTrain":cluster{u16[], u16[]})  [unwired: 6 in]
        }
      }
    }
    frame True {
      w423 = 100.0 ("y")
      n198 = call "BRig_dataLC_ENL_First_OnOff_l1.vi"() -> ("output_ENL_First_OnOff"=w566:i32)  [unwired: 11 in]
      n199 = call "BRig_dataLC_ENL_First_Block_l1.vi"() -> ("output_ENL_First_Block"=w565:i32)  [unwired: 11 in]
      n200 = call "BRig_dataLC_ENL_First_Prob_l1.vi"() -> ("output_ENL_First_Prob"=w564:i32)  [unwired: 11 in]
      n201 = call "BRig_dataLC_ENL_First_Delay_l1.vi"() -> ("output_ENL_First_Delay"=w563:i32)  [unwired: 11 in]
      n202 = call "BRig_dataLC_ENL_First_DelayOpt_l1.vi"() -> ("output_ENL_First_DelayOpt"=w562:i32)  [unwired: 11 in]
      n203 = call "BRig_dataLC_ENL_First_Count_l1.vi"() -> ("output_ENL_First_Count"=w561:i32)  [unwired: 11 in]
      n204 = call "BRig_dataLC_ENL_PreR_OnOff_l1.vi"() -> ("output_ENL_PreR_OnOff"=w560:i32)  [unwired: 11 in]
      n205 = call "BRig_dataLC_ENL_PreR_Block_l1.vi"() -> ("output_ENL_PreR_Block"=w559:i32)  [unwired: 11 in]
      n206 = call "BRig_dataLC_ENL_PreR_Prob_l1.vi"() -> ("output_ENL_PreR_Prob"=w558:i32)  [unwired: 11 in]
      n207 = call "BRig_dataLC_ENL_PreR_Delay_l1.vi"() -> ("output_ENL_PreR_Delay"=w557:i32)  [unwired: 11 in]
      n208 = call "BRig_dataLC_ENL_PreR_DelayOpt_l1.vi"() -> ("output_ENL_PreR_DelayOpt"=w556:i32)  [unwired: 11 in]
      n209 = call "BRig_dataLC_ENL_PreR_Count_l1.vi"() -> ("output_ENL_PreR_Count"=w555:i32)  [unwired: 11 in]
      n210 = call "BRig_dataLC_ENL_PostR_OnOff_l1.vi"() -> ("output_ENL_PostR_OnOff"=w554:i32)  [unwired: 11 in]
      n211 = call "BRig_dataLC_ENL_PostR_Block_l1.vi"() -> ("output_ENL_PostR_Block"=w553:i32)  [unwired: 11 in]
      n212 = call "BRig_dataLC_ENL_PostR_Prob_l1.vi"() -> ("output_ENL_PostR_Prob"=w552:i32)  [unwired: 11 in]
      n213 = call "BRig_dataLC_ENL_PostR_Delay_l1.vi"() -> ("output_ENL_PostR_Delay"=w551:i32)  [unwired: 11 in]
      n214 = call "BRig_dataLC_ENL_PostR_DelayOpt_l1.vi"() -> ("output_ENL_PostR_DelayOpt"=w550:i32)  [unwired: 11 in]
      n215 = call "BRig_dataLC_ENL_PostR_Count_l1.vi"() -> ("output_ENL_PostR_Count"=w549:i32)  [unwired: 11 in]
      n216 = call "BRig_dataLC_ENL2_First_OnOff_l1.vi"() -> ("output_ENL2_First_OnOff"=w408:i32)  [unwired: 11 in]
      n217 = call "BRig_dataLC_ENL2_First_Block_l1.vi"() -> ("output_ENL2_First_Block"=w407:i32)  [unwired: 11 in]
      n218 = call "BRig_dataLC_ENL2_First_Prob_l1.vi"() -> ("output_ENL2_First_Prob"=w406:i32)  [unwired: 11 in]
      n219 = call "BRig_dataLC_ENL2_First_Delay_l1.vi"() -> ("output_ENL2_First_Delay"=w405:i32)  [unwired: 11 in]
      n220 = call "BRig_dataLC_ENL2_First_DelayOpt_l1.vi"() -> ("output_ENL2_First_DelayOpt"=w404:i32)  [unwired: 11 in]
      n221 = call "BRig_dataLC_ENL2_First_Count_l1.vi"() -> ("output_ENL2_First_Count"=w403:i32)  [unwired: 11 in]
      n222 = call "BRig_dataLC_ENL2_PreR_OnOff_l1.vi"() -> ("output_ENL2_PreR_OnOff"=w402:i32)  [unwired: 11 in]
      n223 = call "BRig_dataLC_ENL2_PreR_Block_l1.vi"() -> ("output_ENL2_PreR_Block"=w401:i32)  [unwired: 11 in]
      n224 = call "BRig_dataLC_ENL2_PreR_Prob_l1.vi"() -> ("output_ENL2_PreR_Prob"=w400:i32)  [unwired: 11 in]
      n225 = call "BRig_dataLC_ENL2_PreR_Delay_l1.vi"() -> ("output_ENL2_PreR_Delay"=w399:i32)  [unwired: 11 in]
      n226 = call "BRig_dataLC_ENL2_PreR_DelayOpt_l1.vi"() -> ("output_ENL2_PreR_DelayOpt"=w398:i32)  [unwired: 11 in]
      n227 = call "BRig_dataLC_ENL2_PreR_Count_l1.vi"() -> ("output_ENL2_PreR_Count"=w397:i32)  [unwired: 11 in]
      n228 = call "BRig_dataLC_ENL2_PostR_OnOff_l1.vi"() -> ("output_ENL2_PostR_OnOff"=w396:i32)  [unwired: 11 in]
      n229 = call "BRig_dataLC_ENL2_PostR_Block_l1.vi"() -> ("output_ENL2_PostR_Block"=w395:i32)  [unwired: 11 in]
      n230 = call "BRig_dataLC_ENL2_PostR_Prob_l1.vi"() -> ("output_ENL2_PostR_Prob"=w394:i32)  [unwired: 11 in]
      n231 = call "BRig_dataLC_ENL2_PostR_Delay_l1.vi"() -> ("output_ENL2_PostR_Delay"=w393:i32)  [unwired: 11 in]
      n232 = call "BRig_dataLC_ENL2_PostR_DelayOpt_l1.vi"() -> ("output_ENL2_PostR_DelayOpt"=w392:i32)  [unwired: 11 in]
      n233 = call "BRig_dataLC_ENL2_PostR_Count_l1.vi"() -> ("output_ENL2_PostR_Count"=w391:i32)  [unwired: 11 in]
      n234 = Index Array(array=w445, index #1=w566, index #2=w565, index #3=w564, index #4=w563, index #5=w562, index #6=w561, index #7=w560, index #8=w559, index #9=w558, index #10=w557, index #11=w556, index #12=w555, index #13=w554, index #14=w553, index #15=w552, index #16=w551, index #17=w550, index #18=w549) -> (element #1=w542:u16, element #2=w541:u16, element #3=w540:u16, element #4=w539:u16, element #5=w538:u16, element #6=w537:u16, element #7=w536:u16, element #8=w535:u16, element #9=w534:u16, element #10=w533:u16, element #11=w532:u16, element #12=w531:u16, element #13=w530:u16, element #14=w529:u16, element #15=w528:u16, element #16=w527:u16, element #17=w526:u16, element #18=w525:u16)
      n235 = Index Array(array=w360, index #1=w408, index #2=w407, index #3=w406, index #4=w405, index #5=w404, index #6=w403, index #7=w402, index #8=w401, index #9=w400, index #10=w399, index #11=w398, index #12=w397, index #13=w396, index #14=w395, index #15=w394, index #16=w393, index #17=w392, index #18=w391) -> (element #1=w367:u16, element #2=w368:u16, element #3=w369:u16, element #4=w370:u16, element #5=w371:u16, element #6=w372:u16, element #7=w373:u16, element #8=w374:u16, element #9=w375:u16, element #10=w376:u16, element #11=w377:u16, element #12=w378:u16, element #13=w380:u16, element #14=w381:u16, element #15=w382:u16, element #16=w383:u16, element #17=w384:u16, element #18=w385:u16)
      n236 = Not Equal To 0?(x=w542) -> (x != 0?=w548:bool)
      n237 = Not Equal To 0?(x=w538) -> (x != 0?=w547:bool)
      n238 = Not Equal To 0?(x=w536) -> (x != 0?=w546:bool)
      n239 = Not Equal To 0?(x=w532) -> (x != 0?=w545:bool)
      n240 = Not Equal To 0?(x=w530) -> (x != 0?=w544:bool)
      n241 = Not Equal To 0?(x=w526) -> (x != 0?=w543:bool)
      n242 = local write "LC_ENL_First_OnOff"(w548) -> ()
      n243 = local write "LC_ENL_First_Block"(w541) -> ()
      n244 = local write "LC_ENL_First_Probability"(w540) -> ()
      n245 = local write "LC_ENL_First_Tdelay"(w539) -> ()
      n246 = local write "LC_ENL_First_delayOpt"(w547) -> ()
      n247 = local write "LC_ENL_First_Count"(w537) -> ()
      n248 = local write item#-1(w535) -> ()
      n249 = local write item#-1(w546) -> ()
      n250 = local write item#-1(w531) -> ()
      n251 = local write item#-1(w533) -> ()
      n252 = local write item#-1(w529) -> ()
      n253 = local write item#-1(w544) -> ()
      n254 = local write item#-1(w525) -> ()
      n255 = local write item#-1(w527) -> ()
      n256 = local write item#-1(w545) -> ()
      n257 = local write item#-1(w543) -> ()
      n258 = local write item#-1(w534) -> ()
      n259 = local write item#-1(w528) -> ()
      n260 = Not Equal To 0?(x=w367) -> (x != 0?=w388:bool)
      n261 = Not Equal To 0?(x=w371) -> (x != 0?=w389:bool)
      n262 = Not Equal To 0?(x=w373) -> (x != 0?=w387:bool)
      n263 = Not Equal To 0?(x=w377) -> (x != 0?=w390:bool)
      n264 = Not Equal To 0?(x=w380) -> (x != 0?=w386:bool)
      n265 = Not Equal To 0?(x=w384) -> (x != 0?=w379:bool)
      n266 = call "BRig_dataLC_Cue_PreR_OnOff_l1.vi"() -> ("output_Cue_PreR_OnOff"=w413:i32)  [unwired: 11 in]
      n267 = call "BRig_dataLC_Cue_PreR_Block_l1.vi"() -> ("output_Cue_PreR_Block"=w412:i32)  [unwired: 11 in]
      n268 = call "BRig_dataLC_Cue_PreR_Prob_l1.vi"() -> ("output_Cue_PreR_Prob"=w411:i32)  [unwired: 11 in]
      n269 = call "BRig_dataLC_Cue_PreR_Delay_l1.vi"() -> ("output_Cue_PreR_Delay"=w410:i32)  [unwired: 11 in]
      n270 = call "BRig_dataLC_Cue_PreR_DelayOpt_l1.vi"() -> ("output_Cue_PreR_DelayOpt"=w409:i32)  [unwired: 11 in]
      n271 = call "BRig_dataLC_Cue_PreR_Count_l1.vi"() -> ("output_Cue_PreR_Count"=w414:i32)  [unwired: 11 in]
      n272 = call "BRig_dataLC_Cue_First_OnOff_l1.vi"() -> ("output_Cue_First_OnOff"=w572:i32)  [unwired: 11 in]
      n273 = call "BRig_dataLC_Cue_First_Block_l1.vi"() -> ("output_Cue_First_Block"=w571:i32)  [unwired: 11 in]
      n274 = call "BRig_dataLC_Cue_First_Prob_l1.vi"() -> ("output_Cue_First_Prob"=w570:i32)  [unwired: 11 in]
      n275 = call "BRig_dataLC_Cue_First_Delay_l1.vi"() -> ("output_Cue_First_Delay"=w569:i32)  [unwired: 11 in]
      n276 = call "BRig_dataLC_Cue_First_DelayOpt_l1.vi"() -> ("output_Cue_First_DelayOpt"=w568:i32)  [unwired: 11 in]
      n277 = call "BRig_dataLC_Cue_First_Count_l1.vi"() -> ("output_Cue_First_Count"=w567:i32)  [unwired: 11 in]
      n278 = call "BRig_dataLC_Cue_PostR_OnOff_l1.vi"() -> ("output_Cue_PostR_OnOff"=w419:i32)  [unwired: 11 in]
      n279 = call "BRig_dataLC_Cue_PostR_Block_l1.vi"() -> ("output_Cue_PostR_Block"=w418:i32)  [unwired: 11 in]
      n280 = call "BRig_dataLC_Cue_PostR_Prob_l1.vi"() -> ("output_Cue_PostR_Prob"=w417:i32)  [unwired: 11 in]
      n281 = call "BRig_dataLC_Cue_PostR_Delay_l1.vi"() -> ("output_Cue_PostR_Delay"=w416:i32)  [unwired: 11 in]
      n282 = call "BRig_dataLC_Cue_PostR_DelayOpt_l1.vi"() -> ("output_Cue_PostR_DelayOpt"=w415:i32)  [unwired: 11 in]
      n283 = call "BRig_dataLC_Cue_PostR_Count_l1.vi"() -> ("output_Cue_PostR_Count"=w420:i32)  [unwired: 11 in]
      n284 = local write item#-1(w368) -> ()
      n285 = local write item#-1(w374) -> ()
      n286 = local write item#-1(w388) -> ()
      n287 = local write item#-1(w372) -> ()
      n288 = local write item#-1(w370) -> ()
      n289 = local write item#-1(w387) -> ()
      n290 = local write item#-1(w378) -> ()
      n291 = local write item#-1(w376) -> ()
      n292 = local write item#-1(w381) -> ()
      n293 = local write item#-1(w386) -> ()
      n294 = local write item#-1(w385) -> ()
      n295 = local write item#-1(w383) -> ()
      n296 = local write item#-1(w389) -> ()
      n297 = local write item#-1(w390) -> ()
      n298 = local write item#-1(w369) -> ()
      n299 = local write item#-1(w379) -> ()
      n300 = local write item#-1(w375) -> ()
      n301 = local write item#-1(w382) -> ()
      n302 = call "BRig_dataExp_LED_baseline_Cue.vi"() -> ("output_LED_baseline_Cue"=w444:i32)  [unwired: 11 in]
      n303 = call "BRig_dataExp_L_freq_l1.vi"() -> ("output_L_freq_l1"=w443:i32)  [unwired: 11 in]
      n304 = call "BRig_dataExp_L_T_l1.vi"() -> ("output_L_T_l1"=w442:i32)  [unwired: 11 in]
      n305 = call "BRig_dataExp_L_Tpeak_l1.vi"() -> ("output_L_Tpeak_l1"=w441:i32)  [unwired: 11 in]
      n306 = call "BRig_dataExp_L_Tshutter_l1.vi"() -> ("output_L_Tshutter_l1"=w440:i32)  [unwired: 11 in]
      n307 = call "BRig_dataExp_L_power_min_l1.vi"() -> ("output_L_power_min_l1"=w439:i32)  [unwired: 11 in]
      n308 = call "BRig_dataExp_L_power_max_l1.vi"() -> ("output_L_power_max_l1"=w438:i32)  [unwired: 11 in]
      n309 = call "BRig_dataExp_L_power_step_l1.vi"() -> ("output_L_power_step_l1"=w437:i32)  [unwired: 11 in]
      n310 = Index Array(array=w445, index #1=w572, index #2=w571, index #3=w570, index #4=w569, index #5=w568, index #6=w567, index #7=w413, index #8=w412, index #9=w411, index #10=w410, index #11=w409, index #12=w414, index #13=w419, index #14=w418, index #15=w417, index #16=w416, index #17=w415, index #18=w420) -> (element #1=w518:u16, element #2=w517:u16, element #3=w516:u16, element #4=w515:u16, element #5=w514:u16, element #6=w513:u16, element #7=w512:u16, element #8=w511:u16, element #9=w510:u16, element #10=w509:u16, element #11=w508:u16, element #12=w507:u16, element #13=w506:u16, element #14=w505:u16, element #15=w504:u16, element #16=w503:u16, element #17=w502:u16, element #18=w501:u16)
      n311 = Index Array(array=w360, index #1=w444, index #2=w443, index #3=w442, index #4=w441, index #5=w440, index #6=w439, index #7=w438, index #8=w437) -> (element #1=w436:u16, element #2=w434:u16, element #3=w433:u16, element #4=w432:u16, element #5=w431:u16, element #6=w430:u16, element #7=w429:u16, element #8=w428:u16)
      n312 = To Double Precision Float(number=w430) -> (double precision float=w427:dbl)
      n313 = To Double Precision Float(number=w429) -> (double precision float=w422:dbl)
      n314 = To Double Precision Float(number=w428) -> (double precision float=w421:dbl)
      n315 = Not Equal To 0?(x=w518) -> (x != 0?=w524:bool)
      n316 = Not Equal To 0?(x=w514) -> (x != 0?=w523:bool)
      n317 = Not Equal To 0?(x=w512) -> (x != 0?=w522:bool)
      n318 = Not Equal To 0?(x=w508) -> (x != 0?=w521:bool)
      n319 = Not Equal To 0?(x=w506) -> (x != 0?=w520:bool)
      n320 = Not Equal To 0?(x=w502) -> (x != 0?=w519:bool)
      n321 = Divide(x=w427, y=w423) -> (x/y=w426:dbl)
      n322 = Divide(x=w422, y=w423) -> (x/y=w425:dbl)
      n323 = Divide(x=w421, y=w423) -> (x/y=w424:dbl)
      n324 = local write "LC_Cue_First_OnOff"(w524) -> ()
      n325 = local write "LC_Cue_First_Block"(w517) -> ()
      n326 = local write "LC_Cue_First_Probability"(w516) -> ()
      n327 = local write "LC_Cue_First_Tdelay"(w515) -> ()
      n328 = local write "LC_Cue_First_delayOpt"(w523) -> ()
      n329 = local write "LC_Cue_First_Count"(w513) -> ()
      n330 = Not Equal To 0?(x=w436) -> (x != 0?=w435:bool)
      n331 = call "BRig_dataLC_Cue2_First_OnOff_l1.vi"() -> ("output_Cue2_First_OnOff"=w342:i32)  [unwired: 11 in]
      n332 = call "BRig_dataLC_Cue2_First_Block_l1.vi"() -> ("output_Cue2_First_Block"=w343:i32)  [unwired: 11 in]
      n333 = call "BRig_dataLC_Cue2_First_Prob_l1.vi"() -> ("output_Cue2_First_Prob"=w344:i32)  [unwired: 11 in]
      n334 = call "BRig_dataLC_Cue2_First_Delay_l1.vi"() -> ("output_Cue2_First_Delay"=w345:i32)  [unwired: 11 in]
      n335 = call "BRig_dataLC_Cue2_First_DelayOpt_l1.vi"() -> ("output_Cue2_First_DelayOpt"=w346:i32)  [unwired: 11 in]
      n336 = call "BRig_dataLC_Cue2_First_Count_l1.vi"() -> ("output_Cue2_First_Count"=w347:i32)  [unwired: 11 in]
      n337 = call "BRig_dataLC_Cue2_PreR_OnOff_l1.vi"() -> ("output_Cue2_PreR_OnOff"=w348:i32)  [unwired: 11 in]
      n338 = call "BRig_dataLC_Cue2_PreR_Block_l1.vi"() -> ("output_Cue2_PreR_Block"=w349:i32)  [unwired: 11 in]
      n339 = call "BRig_dataLC_Cue2_PreR_Prob_l1.vi"() -> ("output_Cue2_PreR_Prob"=w350:i32)  [unwired: 11 in]
      n340 = call "BRig_dataLC_Cue2_PreR_Delay_l1.vi"() -> ("output_Cue2_PreR_Delay"=w351:i32)  [unwired: 11 in]
      n341 = call "BRig_dataLC_Cue2_PreR_DelayOpt_l1.vi"() -> ("output_Cue2_PreR_DelayOpt"=w352:i32)  [unwired: 11 in]
      n342 = call "BRig_dataLC_Cue2_PreR_Count_l1.vi"() -> ("output_Cue2_PreR_Count"=w353:i32)  [unwired: 11 in]
      n343 = call "BRig_dataLC_Cue2_PostR_OnOff_l1.vi"() -> ("output_Cue2_PostR_OnOff"=w354:i32)  [unwired: 11 in]
      n344 = call "BRig_dataLC_Cue2_PostR_Block_l1.vi"() -> ("output_Cue2_PostR_Block"=w355:i32)  [unwired: 11 in]
      n345 = call "BRig_dataLC_Cue2_PostR_Prob_l1.vi"() -> ("output_Cue2_PostR_Prob"=w356:i32)  [unwired: 11 in]
      n346 = call "BRig_dataLC_Cue2_PostR_Delay_l1.vi"() -> ("output_Cue2_PostR_Delay"=w357:i32)  [unwired: 11 in]
      n347 = call "BRig_dataLC_Cue2_PostR_DelayOpt_l1.vi"() -> ("output_Cue2_PostR_DelayOpt"=w358:i32)  [unwired: 11 in]
      n348 = call "BRig_dataLC_Cue2_PostR_Count_l1.vi"() -> ("output_Cue2_PostR_Count"=w359:i32)  [unwired: 11 in]
      n349 = local write "LED_baseline"(w435) -> ()
      n350 = local write "Laser_Freq"(w434) -> ()
      n351 = local write "Laser_T"(w433) -> ()
      n352 = local write "Laser_Tpeak"(w432) -> ()
      n353 = local write "Laser_Tshutter"(w431) -> ()
      n354 = local write "Laser_power_min"(w426) -> ()
      n355 = local write "Laser_power_max"(w425) -> ()
      n356 = local write "Laser_power_step"(w424) -> ()
      n357 = local write item#-1(w511) -> ()
      n358 = local write item#-1(w522) -> ()
      n359 = local write item#-1(w507) -> ()
      n360 = local write item#-1(w509) -> ()
      n361 = local write item#-1(w505) -> ()
      n362 = local write item#-1(w520) -> ()
      n363 = local write item#-1(w501) -> ()
      n364 = local write item#-1(w503) -> ()
      n365 = local write item#-1(w521) -> ()
      n366 = local write item#-1(w519) -> ()
      n367 = local write item#-1(w510) -> ()
      n368 = local write item#-1(w504) -> ()
      n369 = Index Array(array=w360, index #1=w342, index #2=w343, index #3=w344, index #4=w345, index #5=w346, index #6=w347, index #7=w348, index #8=w349, index #9=w350, index #10=w351, index #11=w352, index #12=w353, index #13=w354, index #14=w355, index #15=w356, index #16=w357, index #17=w358, index #18=w359) -> (element #1=w361:u16, element #2=w338:u16, element #3=w337:u16, element #4=w336:u16, element #5=w362:u16, element #6=w339:u16, element #7=w363:u16, element #8=w333:u16, element #9=w332:u16, element #10=w331:u16, element #11=w364:u16, element #12=w330:u16, element #13=w365:u16, element #14=w327:u16, element #15=w326:u16, element #16=w325:u16, element #17=w366:u16, element #18=w324:u16)
      n370 = call "BRig_dataLC_Selection_PostR_OnOff_l1.vi"() -> ("output_Selection_PostR_OnOff"=w490:i32)  [unwired: 11 in]
      n371 = call "BRig_dataLC_Selection_PostR_Block_l1.vi"() -> ("output_Selection_PostR_Block"=w489:i32)  [unwired: 11 in]
      n372 = call "BRig_dataLC_Selection_PostR_Prob_l1.vi"() -> ("output_Selection_PostR_Prob"=w488:i32)  [unwired: 11 in]
      n373 = call "BRig_dataLC_Selection_PostR_Delay_l1.vi"() -> ("output_Selection_PostR_Delay"=w487:i32)  [unwired: 11 in]
      n374 = call "BRig_dataLC_Selection_PostR_Count_l1.vi"() -> ("output_Selection_PostR_Count"=w486:i32)  [unwired: 11 in]
      n375 = call "BRig_dataLC_Selection_PreR_OnOff_l1.vi"() -> ("output_Selection_PreR_OnOff"=w495:i32)  [unwired: 11 in]
      n376 = call "BRig_dataLC_Selection_PreR_Block_l1.vi"() -> ("output_Selection_PreR_Block"=w494:i32)  [unwired: 11 in]
      n377 = call "BRig_dataLC_Selection_PreR_Prob_l1.vi"() -> ("output_Selection_PreR_Prob"=w493:i32)  [unwired: 11 in]
      n378 = call "BRig_dataLC_Selection_PreR_Delay_l1.vi"() -> ("output_Selection_PreR_Delay"=w492:i32)  [unwired: 11 in]
      n379 = call "BRig_dataLC_Selection_PreR_Count_l1.vi"() -> ("output_Selection_PreR_Count"=w491:i32)  [unwired: 11 in]
      n380 = call "BRig_dataLC_Selection_First_OnOff_l1.vi"() -> ("output_Selection_First_OnOff"=w500:i32)  [unwired: 11 in]
      n381 = call "BRig_dataLC_Selection_First_Block_l1.vi"() -> ("output_Selection_First_Block"=w499:i32)  [unwired: 11 in]
      n382 = call "BRig_dataLC_Selection_First_Prob_l1.vi"() -> ("output_Selection_First_Prob"=w498:i32)  [unwired: 11 in]
      n383 = call "BRig_dataLC_Selection_First_Delay_l1.vi"() -> ("output_Selection_First_Delay"=w497:i32)  [unwired: 11 in]
      n384 = call "BRig_dataLC_Selection_First_Count_l1.vi"() -> ("output_Selection_First_Count"=w496:i32)  [unwired: 11 in]
      n385 = call "BRig_dataLC_Reward_OnOff_l1.vi"() -> ("output_Reward_OnOff"=w467:i32)  [unwired: 11 in]
      n386 = call "BRig_dataLC_Reward_Block_l1.vi"() -> ("output_Reward_Block"=w466:i32)  [unwired: 11 in]
      n387 = call "BRig_dataLC_Reward_Trial_l1.vi"() -> ("output_Reward_Trial"=w465:i32)  [unwired: 11 in]
      n388 = call "BRig_dataLC_Reward_Prob_l1.vi"() -> ("output_Reward_Prob"=w464:i32)  [unwired: 11 in]
      n389 = call "BRig_dataLC_Reward_Delay_l1.vi"() -> ("output_Reward_Delay"=w463:i32)  [unwired: 11 in]
      n390 = call "BRig_dataLC_Wrong_OnOff_l1.vi"() -> ("output_Wrong_OnOff"=w462:i32)  [unwired: 11 in]
      n391 = call "BRig_dataLC_Wrong_Block_l1.vi"() -> ("output_Wrong_Block"=w461:i32)  [unwired: 11 in]
      n392 = call "BRig_dataLC_Wrong_Trial_l1.vi"() -> ("output_Wrong_Trial"=w460:i32)  [unwired: 11 in]
      n393 = call "BRig_dataLC_Wrong_Prob_l1.vi"() -> ("output_Wrong_Prob"=w459:i32)  [unwired: 11 in]
      n394 = call "BRig_dataLC_Wrong_Delay_l1.vi"() -> ("output_Wrong_Delay"=w458:i32)  [unwired: 11 in]
      n395 = Not Equal To 0?(x=w361) -> (x != 0?=w341:bool)
      n396 = Not Equal To 0?(x=w362) -> (x != 0?=w340:bool)
      n397 = Not Equal To 0?(x=w363) -> (x != 0?=w334:bool)
      n398 = Not Equal To 0?(x=w364) -> (x != 0?=w335:bool)
      n399 = Not Equal To 0?(x=w365) -> (x != 0?=w329:bool)
      n400 = Not Equal To 0?(x=w366) -> (x != 0?=w328:bool)
      n401 = Index Array(array=w445, index #1=w467, index #2=w466, index #3=w465, index #4=w464, index #5=w463, index #6=w462, index #7=w461, index #8=w460, index #9=w459, index #10=w458) -> (element #1=w455:u16, element #2=w454:u16, element #3=w453:u16, element #4=w452:u16, element #5=w451:u16, element #6=w450:u16, element #7=w449:u16, element #8=w448:u16, element #9=w447:u16, element #10=w446:u16)
      n402 = Index Array(array=w445, index #1=w500, index #2=w499, index #3=w498, index #4=w497, index #5=w496, index #6=w495, index #7=w494, index #8=w493, index #9=w492, index #10=w491, index #11=w490, index #12=w489, index #13=w488, index #14=w487, index #15=w486) -> (element #1=w482:u16, element #2=w481:u16, element #3=w480:u16, element #4=w479:u16, element #5=w478:u16, element #6=w477:u16, element #7=w476:u16, element #8=w475:u16, element #9=w474:u16, element #10=w473:u16, element #11=w472:u16, element #12=w471:u16, element #13=w470:u16, element #14=w469:u16, element #15=w468:u16)
      n403 = local write item#-1(w338) -> ()
      n404 = local write item#-1(w333) -> ()
      n405 = local write item#-1(w341) -> ()
      n406 = local write item#-1(w339) -> ()
      n407 = local write item#-1(w336) -> ()
      n408 = local write item#-1(w334) -> ()
      n409 = local write item#-1(w330) -> ()
      n410 = local write item#-1(w331) -> ()
      n411 = local write item#-1(w327) -> ()
      n412 = local write item#-1(w329) -> ()
      n413 = local write item#-1(w324) -> ()
      n414 = local write item#-1(w325) -> ()
      n415 = Not Equal To 0?(x=w455) -> (x != 0?=w457:bool)
      n416 = Not Equal To 0?(x=w450) -> (x != 0?=w456:bool)
      n417 = local write item#-1(w340) -> ()
      n418 = local write item#-1(w335) -> ()
      n419 = local write item#-1(w337) -> ()
      n420 = local write item#-1(w328) -> ()
      n421 = local write item#-1(w332) -> ()
      n422 = local write item#-1(w326) -> ()
      n423 = Not Equal To 0?(x=w482) -> (x != 0?=w485:bool)
      n424 = Not Equal To 0?(x=w477) -> (x != 0?=w484:bool)
      n425 = Not Equal To 0?(x=w472) -> (x != 0?=w483:bool)
      n426 = local write "LC_Reward_OnOff"(w457) -> ()
      n427 = local write "LC_Reward_Block"(w454) -> ()
      n428 = local write "LC_Reward_Probability"(w452) -> ()
      n429 = local write "LC_Reward_Tdelay"(w451) -> ()
      n430 = local write "LC_Sel_First_OnOff"(w485) -> ()
      n431 = local write "LC_Sel_First_Block"(w481) -> ()
      n432 = local write "LC_Sel_First_Probability"(w480) -> ()
      n433 = local write "LC_Sel_First_Tdelay"(w479) -> ()
      n434 = local write "LC_Sel_First_Count"(w478) -> ()
      n435 = local write item#-1(w448) -> ()
      n436 = local write item#-1(w453) -> ()
      n437 = local write item#-1(w449) -> ()
      n438 = local write item#-1(w456) -> ()
      n439 = local write item#-1(w446) -> ()
      n440 = local write item#-1(w447) -> ()
      n441 = local write item#-1(w476) -> ()
      n442 = local write item#-1(w484) -> ()
      n443 = local write item#-1(w473) -> ()
      n444 = local write item#-1(w474) -> ()
      n445 = local write item#-1(w471) -> ()
      n446 = local write item#-1(w483) -> ()
      n447 = local write item#-1(w468) -> ()
      n448 = local write item#-1(w469) -> ()
      n449 = local write item#-1(w475) -> ()
      n450 = local write item#-1(w470) -> ()
    }
  }
  "output_dataLC" <- w4
  "output_dataExp" <- w1
